vi "auger PID.vi"(0 "setpoint":dbl) -> (1 "output":dbl format="%.2f")   [LabVIEW 2012]
uses:
  <vilib>/addons/control/pid/pid.llb/PID (DBL).vi
  <vilib>/addons/control/pid/NI_PID_pid.lvlib
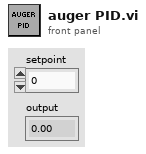
[diagram p1: front panel]
types:
  T1 = cluster{"proportional gain (Kc)":dbl, "integral time (Ti, min)":dbl, "derivative time (Td, min)":dbl}
  T2 = typedef "WPI_EncoderDevRef.ctl" = cluster{"DevStatus":errorcluster, "EncoderIndex":T3, "CounterIndex":T4, "DistancePerCount":dbl, "Decoding Type":T5}
  T3 = typedef "FPGA_EncoderIdx.ctl" = enum8{"Enc 0", "Enc 1", "Enc 2", "Enc 3", "Invalid"}
  T4 = typedef "FPGA_CounterCtrSystemIndex.ctl" = enum8{"Ctr 0", "Ctr 1", "Ctr 2", "Ctr 3", "Ctr 4", "Ctr 5", "Ctr 6", "Ctr 7", "Invalid"}
  T5 = typedef "WPI_EncoderType.ctl" = enum16{"1x", "2x", "4x"}
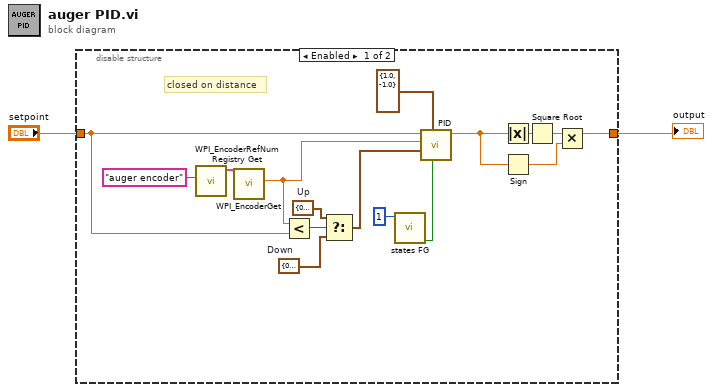
[diagram p0: block diagram]
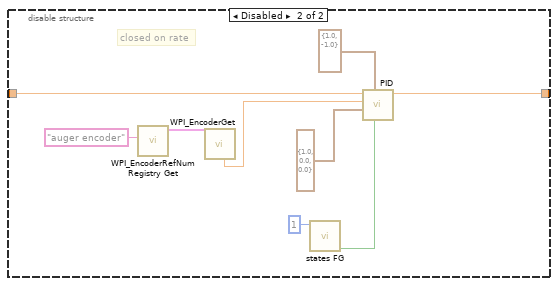
[diagram p2: hidden frame]
diagram:
  n1 = disable-structure shown="Enabled" {
    disable-tunnel: "setpoint" -> [w8 w20]
    disable-tunnel: [w11 w21] -> w1
    frame Enabled {
      w4 = T1 {"proportional gain (Kc)"=0.5, "integral time (Ti, min)"=0.0, "derivative time (Td, min)"=0.0005}  # Down
      w5 = T1 {"proportional gain (Kc)"=0.3, "integral time (Ti, min)"=0.0, "derivative time (Td, min)"=0.0005}  # Up
      # "closed on distance"
      n2 = call <vilib>:"WPI_EncoderRefNum Registry Get.vi"("refnum name"="auger encoder") -> ("EncoderDevRef"=w16:T2)  [unwired: 9 in, 1 out]
      n3 = call <vilib>:"WPI_EncoderGet.vi"("EncoderDevRef"=w16) -> ("Distance"=w7:dbl)  [unwired: 5 in, 5 out]
      n4 = Less?(x=w7, y=w8) -> (x < y?=w6:bool)
      n5 = Select(t=w5, s=w6, f=w4) -> (s? t:f=w3:T1)
      n6 = call "states FG.vi"("Loop ID"=1) -> ("first call?"=w14:bool)  [unwired: 7 in, 3 out]
      n7 = call-poly <vilib>:"PID.vi"("reinitialize? (F)"=w14, "output range"=cluster{"output high":dbl, "output low":dbl} {"output high"=1.0, "output low"=-1.0}, "PID gains"=w3, "process variable"=w7, "setpoint"=w8) -> ("output"=w9:dbl)  [unwired: 5 in, 1 out]
      n8 = Absolute Value(x=w9) -> (abs(x)=w12:dbl)
      n9 = Sign(1:w9) -> (0:w10:dbl)
      n10 = Square Root(x=w12) -> (sqrt(x)=w13:dbl)
      n11 = Multiply(x=w13, y=w10) -> (x*y=w11:dbl)
    }
    frame Disabled {
      # "closed on rate"
      n12 = call <vilib>:"WPI_EncoderRefNum Registry Get.vi"("refnum name"="auger encoder") -> ("EncoderDevRef"=w24:T2)  [unwired: 9 in, 1 out]
      n13 = call <vilib>:"WPI_EncoderGet.vi"("EncoderDevRef"=w24) -> ("Rate"=w19:dbl)  [unwired: 5 in, 5 out]
      n14 = call "states FG.vi"("Loop ID"=1) -> ("first call?"=w22:bool)  [unwired: 7 in, 3 out]
      n15 = call-poly <vilib>:"PID.vi"("reinitialize? (F)"=w22, "output range"=cluster{"output high":dbl, "output low":dbl} {"output high"=1.0, "output low"=-1.0}, "PID gains"=T1 {"proportional gain (Kc)"=1.0, "integral time (Ti, min)"=0.0, "derivative time (Td, min)"=0.0}, "process variable"=w19, "setpoint"=w20) -> ("output"=w21:dbl)  [unwired: 5 in, 1 out]
    }
  }
  "output" <- w1
